vi "Vision Processing.vi"(7 "error out":errorcluster) -> ()   [LabVIEW 2013]
doc: "This VI runs in parallel to other tasks. It gets images from the camera, processes them for color or shape and use that information to affect robot behavior."
uses:
  Robot Global Data.vi
panel:
  out "Numeric":i32
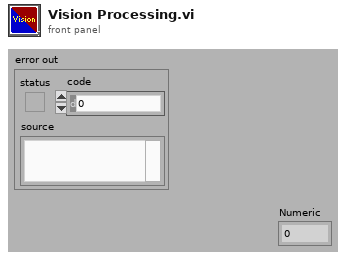
[diagram p1: front panel]
types:
  T1 = cluster{"Target Info 2":cluster{"Center Position":cluster{"X":dbl, "Y":dbl}, "Distance (ft)":dbl, "Center":bool, dbl}[]}
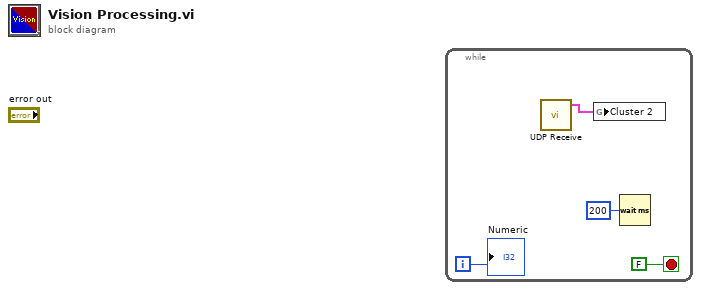
[diagram p0: block diagram]
diagram:
  n1 = while {
    i -> [w3]
    stop <- FALSE stop-if-true
    n2 = call "UDP Receive.vi"() -> ("value"=w1:T1)  [unwired: 5 in]
    n3 = global write "Robot Global Data.vi" "Cluster 2"(w1) -> ()
    n4 = Wait (ms)(milliseconds to wait=u32 200) -> ()  [unwired: 1 out]
    "Numeric" <- w3
  }
